vi "Drive_Cmd_Approach_Camera.vi"(6 "Absolute Angle?":bool, 8 "Absolute Distance?":bool, 9 "Distance":dbl, 10 "Max Power":dbl, 11 "Drive Loop Cluster":T1={"Sensor Data"={"Gyro Data"={"Gyro RT FIFO"=refnum, "Gyro Current"=0.0, "Gyro Hold"=0.0}, "Encoder Data"={"Encoder RT FIFO"=refnum, "Encoder Current"=0.0, "Encoder Hold"=0.0}, "Camera Data"={"Camera RT FIFO"=refnum, "Camera Current"={" Angle"=0.0, "Valid"=FALSE}}}, "PID Update"=refnum, "RobotDriveDevRef"={"DevStatus"={"status"=FALSE, "code"=0, "source"=""}, "Motors[]"=[], "Square Inputs"=FALSE, "Max Output"=1.0}, "Drive Train"=enum."Tank Drive 2 Motor", "Valid Commands"=[], "Drive Comand Notifier"=refnum, "Command Finished?"=refnum, "Command Canceled"=refnum}) -> ()   [LabVIEW 2016]
doc: "Help file writen by FRC Team 836 - The RoboBees\n\nThis VI commands the robot to drive a certain distance.\n\nThis VI writes the \"Drive Distance\" command, power level #3, Distance to travel, and if it is an absoulute angle to the\nDrive Command RT FIFO in Drive Loop Cluster.\n\nThe RT FIFO has to be initialized using the \"Drive_Loop_Initialize_w_Help\" VI"
uses:
  <userlib>/836-libraries/Drive/Drive_Code_V2/Drive_Code_Support/Drive_Code_Bundle.ctl
  <userlib>/836-libraries/Drive/Drive_Code_V2/Drive_Code_Support/SensorTypedefs/Sensor_Cluster.ctl
  <userlib>/836-libraries/Drive/Drive_Code_V2/Drive_Code_Support/SensorTypedefs/Camera_Cluster.ctl
  <userlib>/836-libraries/Drive/Drive_Code_V2/Drive_Code_Support/Drive_Code_PID_Bundle.ctl
  <vilib>/Rock Robotics/WPI/RobotDrive/WPI_RobotDriveDevRef.ctl
  <vilib>/Rock Robotics/WPI/MotorControl/WPI_MotorControlDeviceRef.ctl
  <vilib>/Rock Robotics/WPI/MotorControl/WPI_MotorControlType.ctl
  <vilib>/Rock Robotics/SystemInterfaces/DIO/FPGA_DIOPWMChannel.ctl
  <vilib>/Rock Robotics/WPI/PWM/WPI_PWMDeadband.ctl
  <userlib>/836-libraries/Drive/Drive_Code_V2/Drive_Code_Support/DriveTrains/Drive_Trains.ctl
  <userlib>/836-libraries/Drive/Drive_Code_V2/Drive_Code_Support/Command_Sends/Drive_Code_Command_Type.ctl
  <userlib>/836-libraries/Drive/Drive_Code_V2/Drive_Code_Support/Command_Sends/Drive_Code_Command_List.ctl
  <userlib>/836-libraries/Drive/Drive_Code_V2/Drive_Code_Support/Command_Sends/CommandTypeInfo/ApproachCameraParam.ctl
  <userlib>/836-libraries/Drive/Drive_Code_V2/Drive_Code_Support/Command_Sends/CommandTypeInfo/DistanceInfo.ctl
  <userlib>/836-libraries/Drive/Drive_Code_V2/Drive_Code_Support/Command_Sends/CommandTypeInfo/AngleInfo.ctl
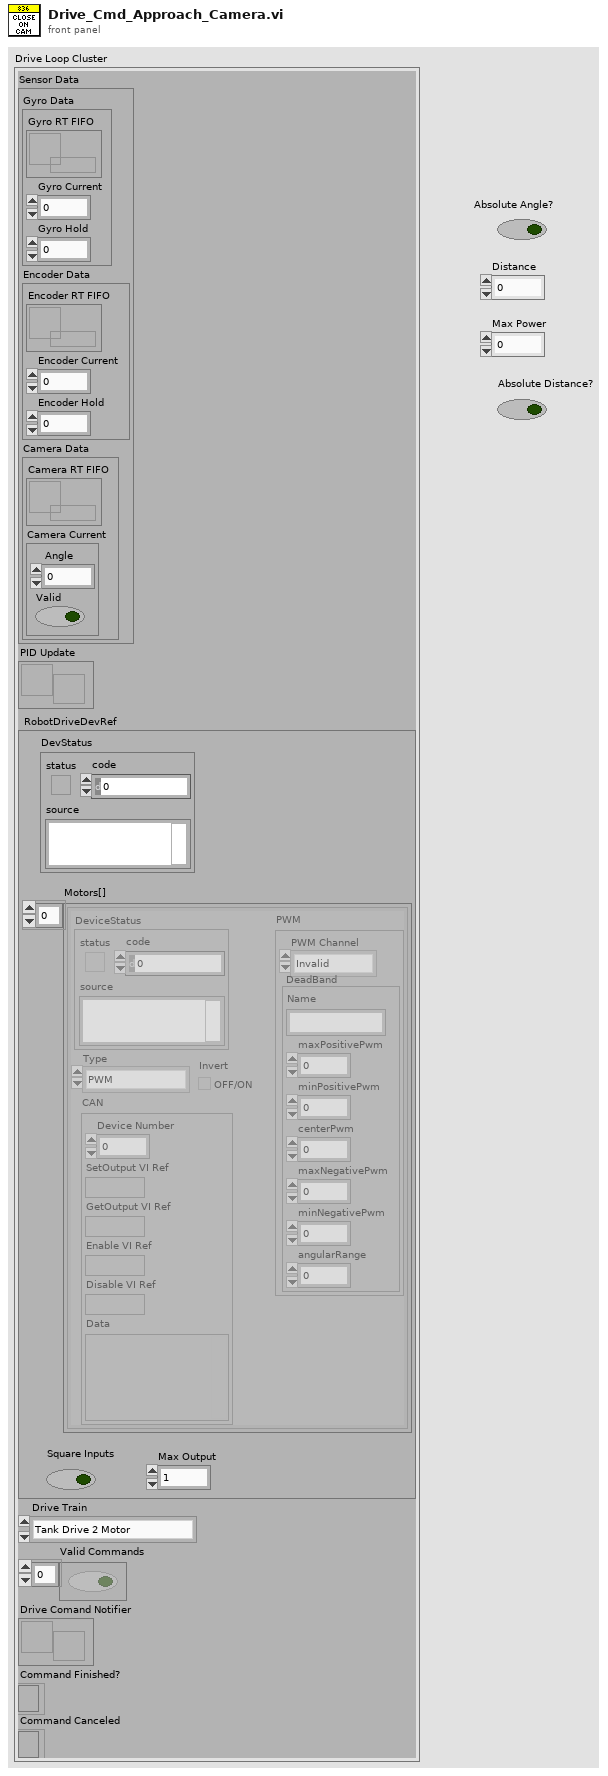
[diagram p1: front panel]
types:
  T1 = typedef "Drive_Code_Bundle.ctl" = cluster{"Sensor Data":T2, "PID Update":refnum<notifier>, "RobotDriveDevRef":T4, "Drive Train":T9, "Valid Commands":bool[], "Drive Comand Notifier":refnum<notifier>, "Command Finished?":refnum<k4>, "Command Canceled":refnum<k4>}
  T2 = typedef "Sensor_Cluster.ctl" = cluster{"Gyro Data":cluster{"Gyro RT FIFO":refnum<k33>, "Gyro Current":dbl, "Gyro Hold":dbl}, "Encoder Data":cluster{"Encoder RT FIFO":refnum<k33>, "Encoder Current":dbl, "Encoder Hold":dbl}, "Camera Data":cluster{"Camera RT FIFO":refnum<k33>, "Camera Current":T3}}
  T3 = typedef "Camera_Cluster.ctl" = cluster{" Angle":dbl, "Valid":bool}
  T4 = typedef "WPI_RobotDriveDevRef.ctl" = cluster{"DevStatus":errorcluster, "Motors[]":T5[], "Square Inputs":bool, "Max Output":dbl}
  T5 = typedef "WPI_MotorControlDeviceRef.ctl" = cluster{"DeviceStatus":errorcluster, "Type":T6, "PWM":cluster{"PWM Channel":T7, "DeadBand":T8}, "CAN":cluster{"Device Number":u8, "SetOutput VI Ref":variant, "GetOutput VI Ref":variant, "Enable VI Ref":variant, "Disable VI Ref":variant, "Data":variant}, "Invert":bool}
  T6 = typedef "WPI_MotorControlType.ctl" = enum16{"PWM", "CAN"}
  T7 = typedef "FPGA_DIOPWMChannel.ctl" = enum8{"PWM 0", "PWM 1", "PWM 2", "PWM 3", "PWM 4", "PWM 5", "PWM 6", "PWM 7", "PWM 8", "PWM 9", "PWM MXP 0", "PWM MXP 1", "PWM MXP 2", "PWM MXP 3", "PWM MXP 4", "PWM MXP 5", "PWM MXP 6", "PWM MXP 7", "PWM MXP 8", "PWM MXP 9", "Invalid"}
  T8 = typedef "WPI_PWMDeadband.ctl" = cluster{"Name":string, "maxPositivePwm":i32, "minPositivePwm":i32, "centerPwm":i32, "maxNegativePwm":i32, "minNegativePwm":i32, "angularRange":u16}
  T9 = typedef "Drive_Trains.ctl" = enum16{"Tank Drive 2 Motor", "Tank Drive 4 Motor", "Mecanum Drive", "Kiwi Drive"}
  T10 = typedef "ApproachCameraParam.ctl" = cluster{"Max Power":dbl, "Distance To Drive":T11, "Angle To Drive At":T12}
  T11 = typedef "DistanceInfo.ctl" = cluster{"Distance":dbl, "Distance Absolute?":bool}
  T12 = typedef "AngleInfo.ctl" = cluster{"Angle":dbl, "Angle Absolute?":bool}
  T13 = typedef "Drive_Code_Command_List.ctl" = enum16{"Do Nothing", "Manual", "Drive Continuous", "Turn", "Drive Distance", "Hold Position", "Hold Yaw", "Follow Camera", "Turn to Camera", "Approach Camera", "PID Update", "Cheesy Drive", "Update Period"}
  T14 = typedef "Drive_Code_Command_Type.ctl" = cluster{"Command":T13, "Command Params":variant}
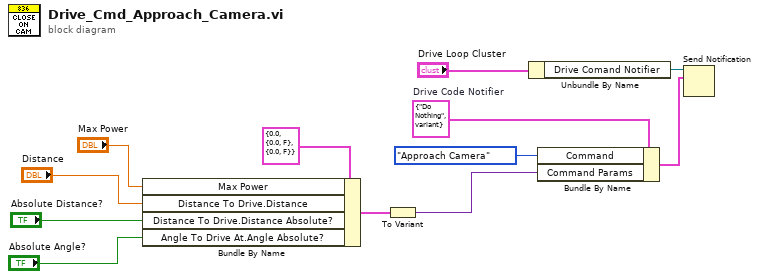
[diagram p0: block diagram]
diagram:
  w8 = T14 {"Command"=enum."Do Nothing", "Command Params"=variant(dbl 0.0)}  # Drive Code Notifier
  n1 = Bundle By Name(cluster=T10 {"Max Power"=0.0, "Distance To Drive"={"Distance"=0.0, "Distance Absolute?"=FALSE}, "Angle To Drive At"={"Angle"=0.0, "Angle Absolute?"=FALSE}} ("Approach Camera Param"), "Max Power"="Max Power", "Distance To Drive.Distance"="Distance", "Distance To Drive.Distance Absolute?"="Absolute Distance?", "Angle To Drive At.Angle Absolute?"="Absolute Angle?") -> (w3:T10)
  n2 = To Variant(anything=w3) -> (Variant=w2:variant)
  n3 = Unbundle By Name("Drive Loop Cluster") -> ("Drive Comand Notifier"=w12:refnum<notifier>)
  n4 = Bundle By Name(cluster=w8, "Command"=Drive_Code_Command_List."Approach Camera", "Command Params"=w2) -> (w11:T14)
  n5 = Send Notification(notification=w11, notifier=w12) -> ()  [unwired: 1 in, 2 out]
